vi "TIFF Get Tag List Entry.vi"(8 "error in (no error)":errorcluster, 10 "tag_index":cluster{}, 11 "para0":cluster{}) -> (0 "error out":errorcluster, 2 "function return":u32, 3 "para0 out":cluster{})   [LabVIEW 2018]
doc: "LIBTIFF_DLL_IMPEXP ttag_t TIFFGetTagListEntry( TIFF *, int tag_index );\nextern ttag_t TIFFGetTagListEntry( TIFF *, int tag_index );"
uses:
  libtiff3.dll
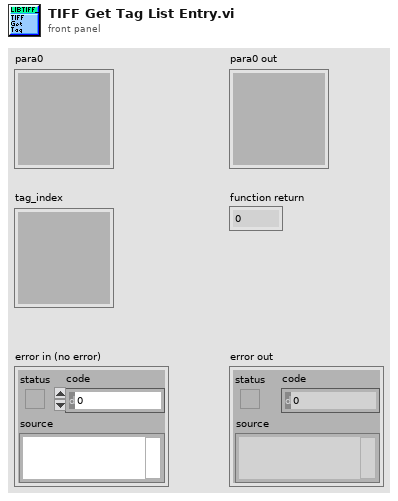
[diagram p1: front panel]
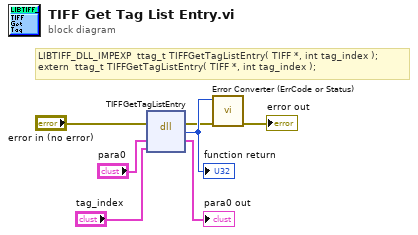
[diagram p0: block diagram]
diagram:
  # "LIBTIFF_DLL_IMPEXP  ttag_t TIFFGetTagListEntry( TIFF *, int tag_index );\nextern  ttag_t TIFFGetTagListEntry( TIFF *, int tag_index );"
  n1 = dll-call lib="C:/Users/johan/Downloads/LabVIEW software/LabVIEW software/IX-81 Software/lib/tiff/LibTiffLabview/libtiff3.*" fn="TIFFGetTagListEntry"(error in="error in (no error)", "para0"="para0", "tag_index"="tag_index") -> (error out=w2:errorcluster, w7:u32, "para0"=→"para0 out":cluster{})  [unwired: 3 in, 1 out]
  "function return" <- w7
  n2 = call "Error Converter (ErrCode or Status).vi"("error in (no error)"=w2, "error code"=w7) -> ("error out"=→"error out":errorcluster)  [unwired: 9 in]
